vi "creatbuf.vi"(7 "DigitizerIdVarPtr":refnum<k24>, 8 "SystemIdVarPtr":refnum<k24>, 9 ".NET  in":refnum<k24>) -> (0 "w":i32, 1 "h":i32, 2 "MbufAlloc2d":refnum<k24>, 3 ".NET  out":refnum<k24>)   [LabVIEW 2019]
uses:
  C:/Users/huang/Desktop/MIL LITE 10/64/Matrox Imaging/MIL/MIL.NET/Matrox.MatroxImagingLibrary.v3.5.dll
  64/Matrox Imaging/MIL/MIL.NET/Matrox.MatroxImagingLibrary.v3.5.dll
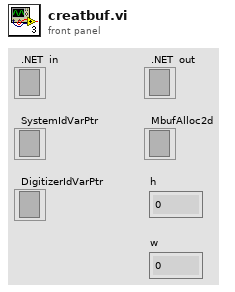
[diagram p1: front panel]
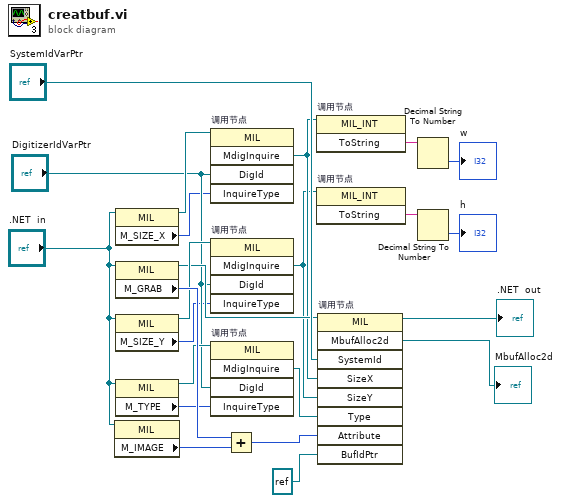
[diagram p0: block diagram]
diagram:
  n1 = property class="MIL"(reference=".NET  in") -> ("M_IMAGE"=w22:i32)  [unwired: 1 in, 2 out]
  n2 = property class="MIL"(reference=".NET  in") -> (reference out=w19:refnum<k24>, "M_SIZE_X"=w9:i32)  [unwired: 1 in, 1 out]
  n3 = property class="MIL"(reference=".NET  in") -> (reference out=w13:refnum<k24>, "M_GRAB"=w23:i32)  [unwired: 1 in, 1 out]
  n4 = property class="MIL"(reference=".NET  in") -> (reference out=w20:refnum<k24>, "M_SIZE_Y"=w8:i32)  [unwired: 1 in, 1 out]
  n5 = property class="MIL"(reference=".NET  in") -> (reference out=w18:refnum<k24>, "M_TYPE"=w17:i32)  [unwired: 1 in, 1 out]
  n6 = invoke on="调用节点" class="MIL" method="MdigInquire"(reference=w19, "DigId"="DigitizerIdVarPtr", "InquireType"=w9) -> ("MdigInquire"=w7:refnum<k24>)  [unwired: 2 in, 4 out]
  n7 = invoke on="调用节点" class="MIL" method="MdigInquire"(reference=w20, "DigId"="DigitizerIdVarPtr", "InquireType"=w8) -> ("MdigInquire"=w4:refnum<k24>)  [unwired: 2 in, 4 out]
  n8 = invoke on="调用节点" class="MIL" method="MdigInquire"(reference=w18, "DigId"="DigitizerIdVarPtr", "InquireType"=w17) -> ("MdigInquire"=w16:refnum<k24>)  [unwired: 2 in, 4 out]
  n9 = Add(x=w23, y=w22) -> (x+y=w14:i32)
  n10 = invoke on="调用节点" class="MIL_INT" method="ToString"(reference=w7) -> ("ToString"=w6:string)  [unwired: 2 in, 2 out]
  n11 = invoke on="调用节点" class="MIL_INT" method="ToString"(reference=w4) -> ("ToString"=w3:string)  [unwired: 2 in, 2 out]
  n12 = invoke on="调用节点" class="MIL" method="MbufAlloc2d"(reference=w13, "SystemId"="SystemIdVarPtr", "SizeX"=w7, "SizeY"=w4, "Type"=w16, "Attribute"=w14, "BufIdPtr"=refnum<k24> refnum) -> (reference out=→".NET  out":refnum<k24>, "MbufAlloc2d"=→"MbufAlloc2d":refnum<k24>)  [unwired: 2 in, 7 out]
  n13 = Decimal String To Number(string=w6) -> (number=→"w":i32)  [unwired: 2 in, 1 out]
  n14 = Decimal String To Number(string=w3) -> (number=→"h":i32)  [unwired: 2 in, 1 out]
